vi "对称性补点.vi"(10 "检测点":dbl[](array[numeric]), 11 "XY图":cluster{dbl[], dbl[]}[](graph)) -> (2 "回正率":dbl[](array[numeric]), 3 "对称性":dbl[](array[numeric]))   [LabVIEW 2020]
uses:
  <vilib>/Analysis/NI_AAL_Geometry.lvlib
panel:
  out "右1":dbl[](array[numeric])
  out "左1":dbl[](array[numeric])
  out "右":dbl[](array[numeric])
  out "左":dbl[](array[numeric])
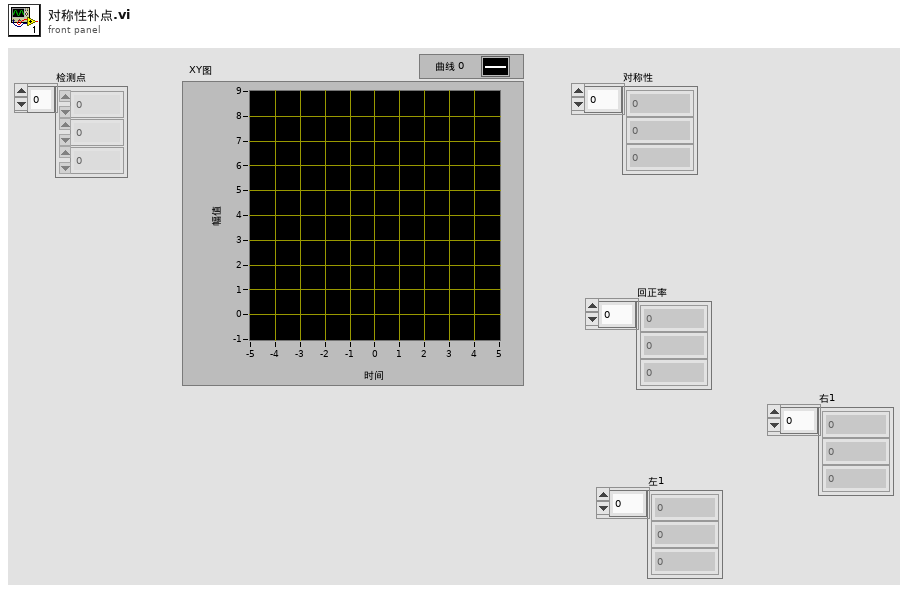
[diagram p1: front panel]
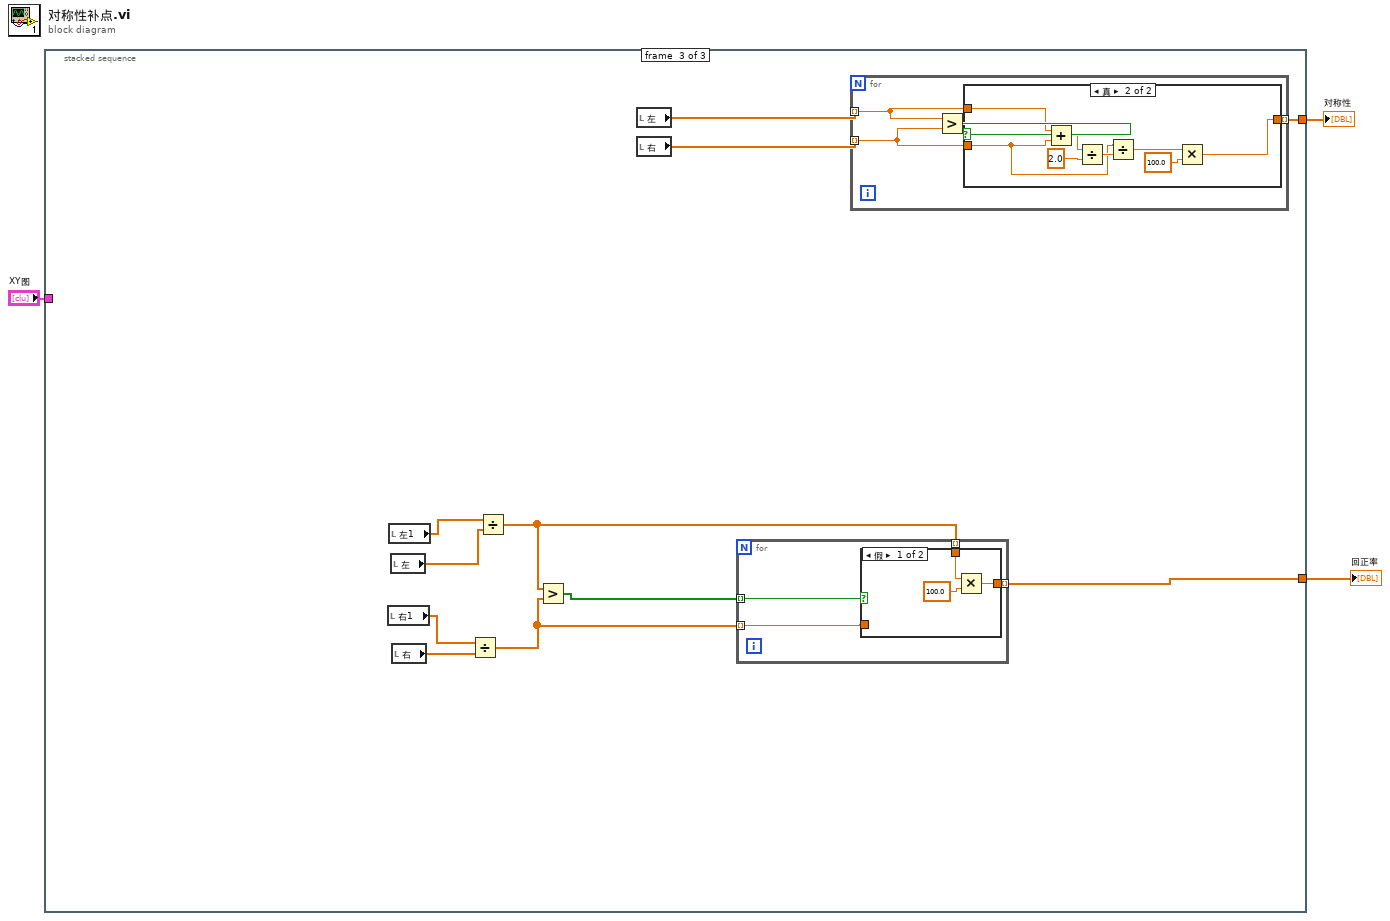
[diagram p0: block diagram]
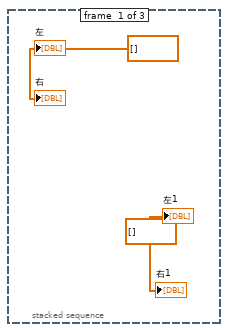
[diagram p2: hidden frame]
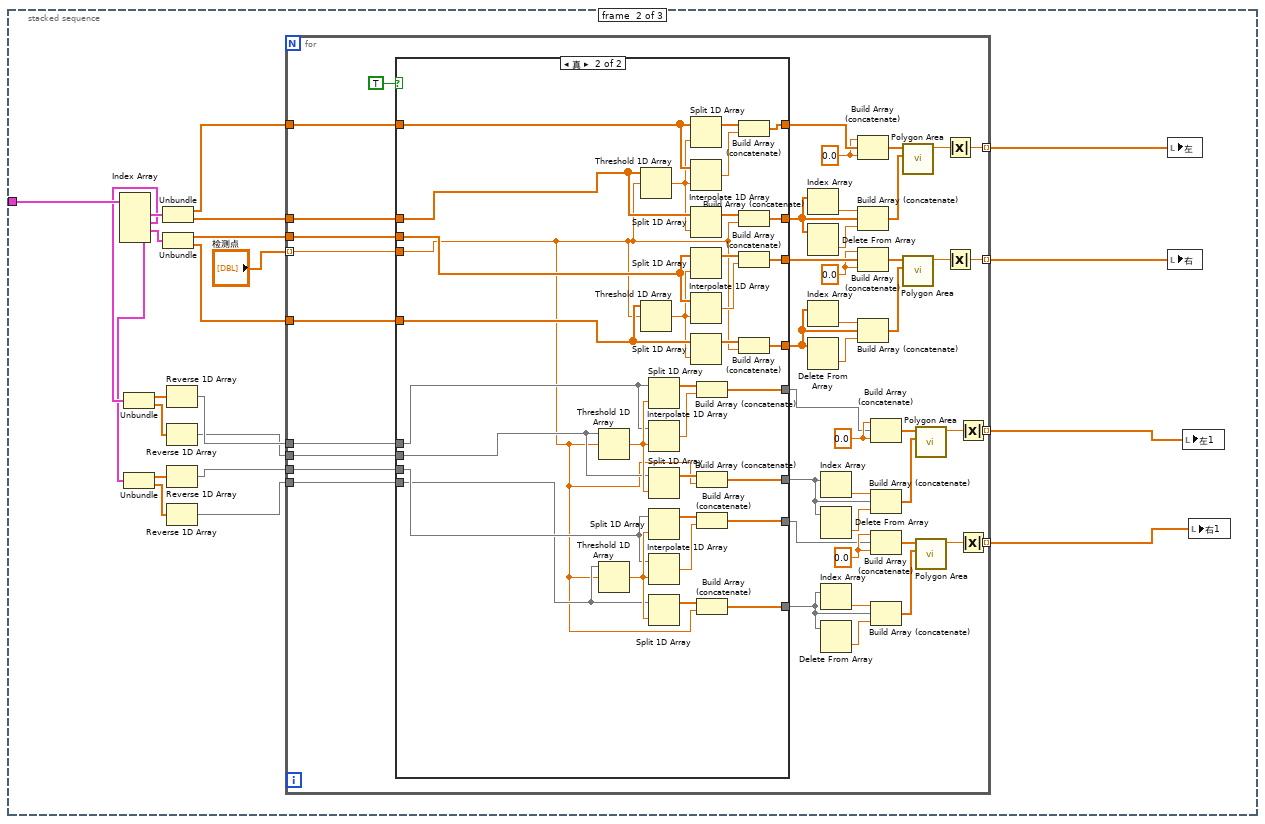
[diagram p3: hidden frame]
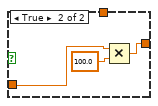
[diagram p5: hidden frame]
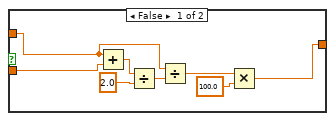
[diagram p6: hidden frame]
diagram:
  n1 = stacked-sequence {
    tunnel: "XY图" -> [_ w27 _]
    tunnel: [_ _ w115] -> w3
    tunnel: [_ _ w118] -> w1
    frame #0 {
      w4 = dbl[] [] ("左")
      w5 = dbl[] [] ("左")
      "左" <- w5
      "右" <- w5
      "右1" <- w4
      "左1" <- w4
    }
    frame #1 {
      n2 = Index Array(array=w27) -> (element #1=w20:cluster{dbl[], dbl[]}, element #2=w17:cluster{dbl[], dbl[]}, element #3=w18:cluster{dbl[], dbl[]}, element #4=w16:cluster{dbl[], dbl[]})  [unwired: 4 in]
      n3 = Unbundle(w17) -> (w13:dbl[], w11:dbl[])
      n4 = Unbundle(w16) -> (w9:dbl[], w7:dbl[])
      n5 = Unbundle(w20) -> (w26:dbl[], w23:dbl[])
      n6 = Unbundle(w18) -> (w24:dbl[], w25:dbl[])
      n7 = Reverse 1D Array(array=w13) -> (reversed array=w12:dbl[])
      n8 = Reverse 1D Array(array=w11) -> (reversed array=w10:dbl[])
      n9 = Reverse 1D Array(array=w9) -> (reversed array=w8:dbl[])
      n10 = Reverse 1D Array(array=w7) -> (reversed array=w6:dbl[])
      n11 = for {
        tunnel: w26 -> [w71]
        tunnel: w25 -> [w70]
        tunnel: w24 -> [w69]
        tunnel: w23 -> [w68]
        tunnel: [w58] -> w22 mode=indexing
        tunnel: [w57] -> w21 mode=indexing
        tunnel: "检测点" -> [w50] mode=indexing
        tunnel: w12 -> [w49]
        tunnel: w8 -> [w48]
        tunnel: w10 -> [w47]
        tunnel: w6 -> [w46]
        tunnel: [w29] -> w15 mode=indexing
        tunnel: [w28] -> w14 mode=indexing
        w36 = 0.0
        w37 = 0.0
        w53 = 0.0
        w54 = 0.0
        n12 = case shown="真" TRUE {
          tunnel: w71 -> [w81 w107]
          tunnel: w70 -> [w78 w113]
          tunnel: w69 -> [w79 w102]
          tunnel: w68 -> [w80 w114]
          tunnel: [w81 w108] -> w67
          tunnel: [w80 w104] -> w65
          tunnel: [w78 w99] -> w61
          tunnel: [w79 w103] -> w60
          tunnel: w50 -> [_ w86]
          tunnel: w49 -> [w77 w90]
          tunnel: w48 -> [w75 w88]
          tunnel: w47 -> [w76 w89]
          tunnel: w46 -> [w74 w87]
          tunnel: [w77 w85] -> w33
          tunnel: [w76 w84] -> w32
          tunnel: [w75 w83] -> w31
          tunnel: [w74 w82] -> w30
          frame False {
          }
          frame True {
            n13 = Threshold 1D Array(2:w86, 3:w89) -> (0:w94:dbl)  [unwired: 1 in]
            n14 = Threshold 1D Array(2:w86, 3:w87) -> (0:w92:dbl)  [unwired: 1 in]
            n15 = Threshold 1D Array(2:w86, 3:w114) -> (0:w106:dbl)  [unwired: 1 in]
            n16 = Threshold 1D Array(2:w86, 3:w113) -> (0:w101:dbl)  [unwired: 1 in]
            n17 = Split 1D Array(array=w90, index=w94) -> (first subarray=w98:dbl[])  [unwired: 1 out]
            n18 = Interpolate 1D Array(1:w94, 2:w90) -> (0:w93:dbl)
            n19 = Split 1D Array(array=w89, index=w94) -> (first subarray=w97:dbl[])  [unwired: 1 out]
            n20 = Split 1D Array(array=w88, index=w92) -> (first subarray=w95:dbl[])  [unwired: 1 out]
            n21 = Interpolate 1D Array(1:w92, 2:w88) -> (0:w91:dbl)
            n22 = Split 1D Array(array=w87, index=w92) -> (first subarray=w96:dbl[])  [unwired: 1 out]
            n23 = Split 1D Array(array=w107, index=w106) -> (first subarray=w112:dbl[])  [unwired: 1 out]
            n24 = Interpolate 1D Array(1:w106, 2:w107) -> (0:w105:dbl)
            n25 = Split 1D Array(array=w114, index=w106) -> (first subarray=w111:dbl[])  [unwired: 1 out]
            n26 = Split 1D Array(array=w102, index=w101) -> (first subarray=w109:dbl[])  [unwired: 1 out]
            n27 = Interpolate 1D Array(1:w101, 2:w102) -> (0:w100:dbl)
            n28 = Split 1D Array(array=w113, index=w101) -> (first subarray=w110:dbl[])  [unwired: 1 out]
            n29 = Build Array (concatenate)(w98, w93) -> (w85:dbl[])
            n30 = Build Array (concatenate)(w97, w86) -> (w84:dbl[])
            n31 = Build Array (concatenate)(w95, w91) -> (w83:dbl[])
            n32 = Build Array (concatenate)(w96, w86) -> (w82:dbl[])
            n33 = Build Array (concatenate)(w112, w105) -> (w108:dbl[])
            n34 = Build Array (concatenate)(w111, w86) -> (w104:dbl[])
            n35 = Build Array (concatenate)(w109, w100) -> (w103:dbl[])
            n36 = Build Array (concatenate)(w110, w86) -> (w99:dbl[])
          }
        }
        n37 = Index Array(array=w65) -> (element=w66:dbl)  [unwired: 1 in]
        n38 = Delete From Array(array=w65) -> (deleted portion=w64:dbl)  [unwired: 2 in, 1 out]
        n39 = Index Array(array=w61) -> (element=w62:dbl)  [unwired: 1 in]
        n40 = Delete From Array(array=w61) -> (deleted portion=w63:dbl)  [unwired: 2 in, 1 out]
        n41 = Index Array(array=w32) -> (element=w43:dbl)  [unwired: 1 in]
        n42 = Delete From Array(array=w32) -> (deleted portion=w42:dbl)  [unwired: 2 in, 1 out]
        n43 = Index Array(array=w30) -> (element=w40:dbl)  [unwired: 1 in]
        n44 = Delete From Array(array=w30) -> (deleted portion=w41:dbl)  [unwired: 2 in, 1 out]
        n45 = Build Array (concatenate)(w54, w67, w54) -> (w56:dbl[])
        n46 = Build Array (concatenate)(w66, w65, w64) -> (w51:dbl[])
        n47 = Build Array (concatenate)(w53, w60, w53) -> (w52:dbl[])
        n48 = Build Array (concatenate)(w62, w61, w63) -> (w55:dbl[])
        n49 = Build Array (concatenate)(w37, w33, w37) -> (w39:dbl[])
        n50 = Build Array (concatenate)(w43, w32, w42) -> (w34:dbl[])
        n51 = Build Array (concatenate)(w36, w31, w36) -> (w35:dbl[])
        n52 = Build Array (concatenate)(w40, w30, w41) -> (w38:dbl[])
        n53 = call <vilib>:"Polygon Area.vi"("Y"=w51, "X"=w56) -> ("signed area"=w72:dbl)  [unwired: 8 in, 1 out]
        n54 = call <vilib>:"Polygon Area.vi"("Y"=w55, "X"=w52) -> ("signed area"=w73:dbl)  [unwired: 8 in, 1 out]
        n55 = call <vilib>:"Polygon Area.vi"("Y"=w34, "X"=w39) -> ("signed area"=w44:dbl)  [unwired: 8 in, 1 out]
        n56 = call <vilib>:"Polygon Area.vi"("Y"=w38, "X"=w35) -> ("signed area"=w45:dbl)  [unwired: 8 in, 1 out]
        n57 = Absolute Value(x=w72) -> (abs(x)=w58:dbl)
        n58 = Absolute Value(x=w73) -> (abs(x)=w57:dbl)
        n59 = Absolute Value(x=w44) -> (abs(x)=w29:dbl)
        n60 = Absolute Value(x=w45) -> (abs(x)=w28:dbl)
      }
      n61 = local write "左"(w22) -> ()
      n62 = local write "右"(w21) -> ()
      n63 = local write "左1"(w15) -> ()
      n64 = local write "右1"(w14) -> ()
    }
    frame #2 {
      n65 = local read "右1"() -> (w121:dbl[])
      n66 = local read "左1"() -> (w123:dbl[])
      n67 = local read "左"() -> (w122:dbl[])
      n68 = local read "右"() -> (w120:dbl[])
      n69 = Divide(x=w121, y=w120) -> (x/y=w117:dbl[])
      n70 = Divide(x=w123, y=w122) -> (x/y=w116:dbl[])
      n71 = Greater?(x=w116, y=w117) -> (0:w119:bool[])
      n72 = local read "左"() -> (w124:dbl[])
      n73 = local read "右"() -> (w125:dbl[])
      n74 = for {
        tunnel: [w129] -> w118 mode=indexing
        tunnel: w119 -> [w128] mode=indexing
        tunnel: w117 -> [w127] mode=indexing
        tunnel: w116 -> [w126] mode=indexing
        n75 = case shown="假" w128 {
          tunnel: [w131 w135] -> w129
          tunnel: w127 -> [_ w133]
          tunnel: w126 -> [w130 _]
          frame False {
            n76 = Multiply(x=w130, y=100.0) -> (x*y=w131:dbl)
          }
          frame True {
            n77 = Multiply(x=w133, y=100.0) -> (x*y=w135:dbl)
          }
        }
      }
      n78 = for {
        tunnel: w125 -> [w136] mode=indexing
        tunnel: w124 -> [w138] mode=indexing
        tunnel: [w137] -> w115 mode=indexing
        n79 = Greater?(x=w138, y=w136) -> (0:w139:bool)
        n80 = case shown="真" w139 {
          tunnel: w138 -> [w141 w149]
          tunnel: [w142 w150] -> w137
          tunnel: w136 -> [w140 w148]
          frame False {
            n81 = Add(x=w141, y=w140) -> (x+y=w145:dbl)
            n82 = Divide(x=w145, y=2.0) -> (x/y=w143:dbl)
            n83 = Divide(x=w141, y=w143) -> (x/y=w147:dbl)
            n84 = Multiply(x=w147, y=100.0) -> (x*y=w142:dbl)
          }
          frame True {
            n85 = Add(x=w149, y=w148) -> (x+y=w153:dbl)
            n86 = Divide(x=w153, y=2.0) -> (x/y=w151:dbl)
            n87 = Divide(x=w148, y=w151) -> (x/y=w155:dbl)
            n88 = Multiply(x=w155, y=100.0) -> (x*y=w150:dbl)
          }
        }
      }
    }
  }
  "对称性" <- w3
  "回正率" <- w1
